vi "tcp_server_connect.vi"(8 "error in":errorcluster, 10 "Config":T1={"IO params"={"Conversion"={"Rate"=4.0, "Num cards"=2, "Out channels"=4}, "Carriers"={"Phase shift"=180.0, "Levels"=[[0.8, 0.8, 0.8], [0.03, 0.03, 0.03]], "Delay samples"=73.15}, "TCP"={"Host"="192.168.1.15", "Port"=6666, "Buffering"=6, "Timeout"=6}}, "High rate STFT"={"Win param"=101.5, "Window type"=61, "Win order"=2, "DFT size"=64, "Channels"=[7], "Oversample"=64}, "Low rate STFT"={"Win param"=120.0, "Window type"=61, "Win order"=8, "DFT size"=64, "Channels"=[7], "Oversample"=64}, "Filtering "=[]} {"Filtering"."Distortion"."Limit" format="%#_3p"; "Filtering"."Distortion"."LF cut" format="%#_3p"; "Filtering"."Kalman"."Measure noise" format="%#_3p"; "Filtering"."Kalman"."Process noise" format="%#_3p"; "Filtering"."Hum"."Limit" format="%#_3p"; "Filtering"."Hum"."Frequency" format="%#_4p"; "Low rate STFT"."Oversample" min=1 step=1; "Low rate STFT"."Channels" min=0 step=1; "Low rate STFT"."DFT size" min=1 step=1; "Low rate STFT"."Window type" items=["Rectangle"=0, "Hanning"=1, "Hamming"=2, "Blackman-Harris"=3, "Exact Blackman"=4, "Blackman"=5, "Flat Top"=6, "4 Term B-Harris "=7, "7 Term B-Harris"=8, "Low Sidelobe"=9, "Blackman Nuttall"=11, "Triangle"=30, "Bartlett-Hanning"=31, "Bohman"=32, "Parzen"=33, "Welch"=34, "Kaiser"=60, "Dolph-Chebyshev"=61, "Gaussian"=62]; "High rate STFT"."Oversample" min=1 step=1; "High rate STFT"."Channels" min=0 step=1; "High rate STFT"."DFT size" min=1 step=1; "High rate STFT"."Window type" items=["Rectangle"=0, "Hanning"=1, "Hamming"=2, "Blackman-Harris"=3, "Exact Blackman"=4, "Blackman"=5, "Flat Top"=6, "4 Term B-Harris "=7, "7 Term B-Harris"=8, "Low Sidelobe"=9, "Blackman Nuttall"=11, "Triangle"=30, "Bartlett-Hanning"=31, "Bohman"=32, "Parzen"=33, "Welch"=34, "Kaiser"=60, "Dolph-Chebyshev"=61, "Gaussian"=62]; "IO params"."Carriers"."Levels" min=0.0 step=0.1; "IO params"."Conversion"."Rate" format="%#_8g"}) -> (0 "error out":errorcluster, 3 "connection ID":refnum<k5>)   [LabVIEW 2014]
uses:
  processing/ilemt_config.ctl
  IO_params.ctl
  processing/stft_params.ctl
  <vilib>/Analysis/4window.llb/windowTd.ctl
  processing/filter_params.ctl
  processing/detrend_mode.ctl
  <vilib>/Analysis/NI_AALPro.lvlib
panel:
  in  "Open count":i32
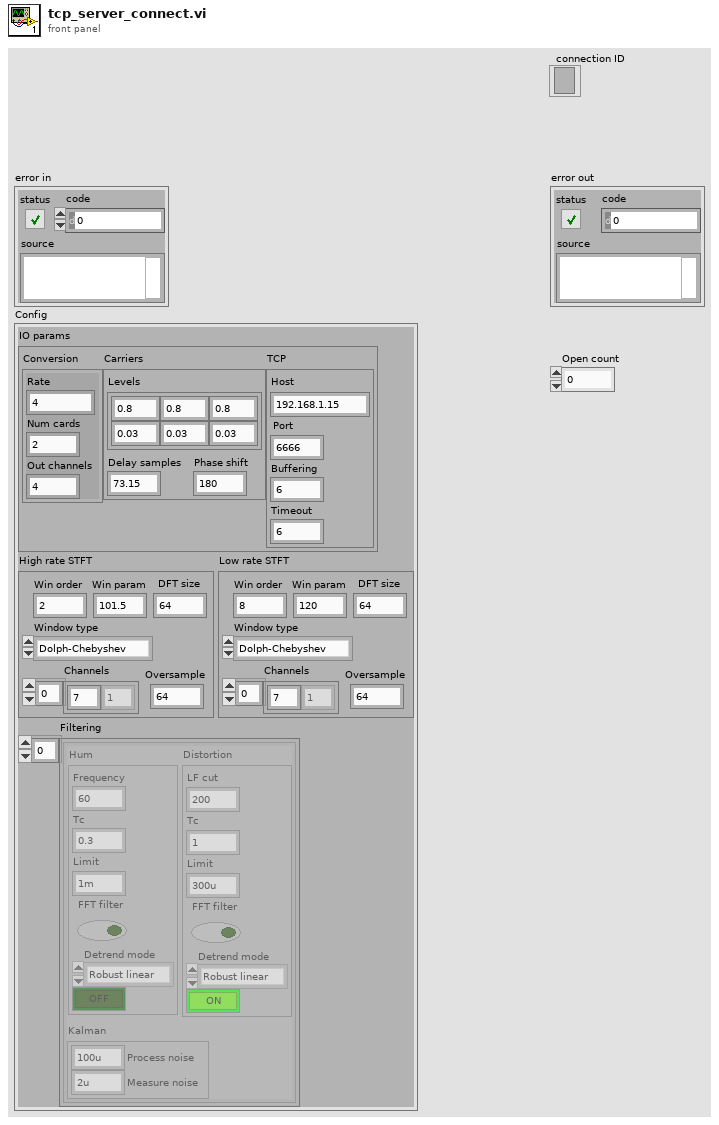
[diagram p1: front panel]
types:
  T1 = typedef "ilemt_config.ctl" = cluster{"IO params":T2, "High rate STFT":T3, "Low rate STFT":T3, "Filtering ":T5[]}
  T2 = typedef "IO_params.ctl" = cluster{"Conversion":cluster{"Rate":dbl, "Num cards":u32, "Out channels":u32}, "Carriers":cluster{"Phase shift":dbl, "Levels":dbl[][], "Delay samples":dbl}, "TCP":cluster{"Host":string, "Port":i32, "Buffering":u32, "Timeout":u32}}
  T3 = typedef "stft_params.ctl" = cluster{"Win param":dbl, "Window type":T4, "Win order":i32, "DFT size":i32, "Channels":i32[], "Oversample":i32}
  T4 = typedef "NI_AALPro.lvlib/windowTd.ctl" = u32
  T5 = typedef "filter_params.ctl" = cluster{"Hum":cluster{"Frequency":dbl, "Tc":dbl, "Limit":dbl, "FFT filter":bool, "Detrend mode":T6, "Enable":bool}, "Kalman":cluster{"Process noise":dbl, "Measure noise":dbl}, "Distortion":cluster{"LF cut":dbl, "Tc":dbl, "Limit":dbl, "FFT filter":bool, "Detrend mode":T6, "Enable":bool}}
  T6 = typedef "detrend_mode.ctl" = enum16{"Zero mean", "Linear", "Robust linear"}
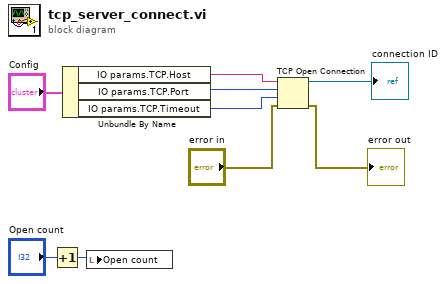
[diagram p0: block diagram]
diagram:
  n1 = Increment(x="Open count") -> (x+1=w2:i32)
  n2 = Unbundle By Name("Config") -> ("IO params.TCP.Host"=w6:string, "IO params.TCP.Port"=w5:i32, "IO params.TCP.Timeout"=w1:u32)
  n3 = local write "Open count"(w2) -> ()
  n4 = TCP Open Connection(address=w6, remote port or service name=w5, timeout ms (60000)=w1, error in (no error)="error in") -> (connection ID=→"connection ID":refnum<k5>, error out=→"error out":errorcluster)  [unwired: 1 in]
